vi "ResetTCPCommands&Responses_GIS Printer.vi"(8 "error in (no error)":errorcluster, 11 "GIS Printer In":refnum<class "GIS Printer.lvclass">) -> (0 "error out":errorcluster, 3 "GIS Printer Out":refnum<class "GIS Printer.lvclass">)   [LabVIEW 2022 SP3, in "GIS Printer.lvclass"]
uses:
  GIS Printer.lvclass
  GIS Printer.lvclass/GIS Printer.ctl
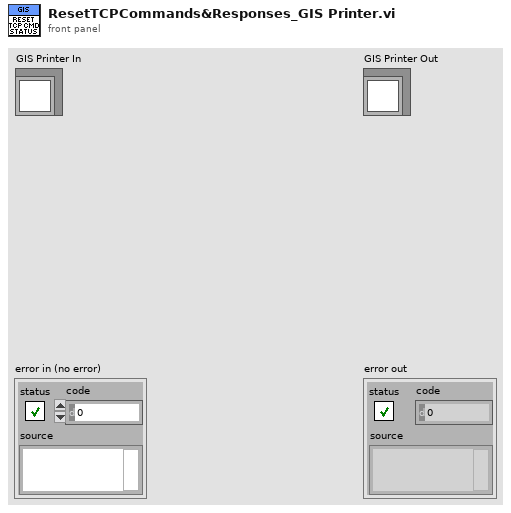
[diagram p1: front panel]
types:
  T1 = typedef "GIS Printer.lvclass/Private Data.ctl" = cluster{"UserEvents":T2, "All Dependencies":cluster{"Class References":refnum<class>[], "Class Names":string[]}, "PrinterConiguration":T3, "Status":T4, "GISHeadStatus":T5[], "HeadStatus":T6}
  T2 = typedef "GIS Printer.lvclass/UserEvents.ctl" = cluster{"API Incoming Event":refnum<user-event>, "API Executed Event":refnum<user-event>, "API Return Event":refnum<user-event>, "Status Changed Event":refnum<user-event>, "Abort":refnum<user-event>, "stop process":refnum<user-event>, "GISPollStatus":refnum<user-event>, "GISHeadStatus":refnum<user-event>}
  T3 = typedef "GIS Printer.lvclass/PrinterConfiguration--Cluster.ctl" = cluster{"IPAddress":string, "Move Stage on RTP Command?":bool, "Stage Move Position":string, "PH1-Prime Path":path, "PH2-Prime Path":path, "PH3-Prime Path":path, "PH4-Prime Path":path, "PH5-Prime Path":path, "PH6-Prime Path":path, "PrintScriptsFolder":path, "PurgeScriptsFolder":path, "StageScriptsFolder":path, "PH1-HeatOn Path":path, "PH2-HeatOn Path":path, "PH3-HeatOn Path":path, "PH4-HeatOn Path":path, "PH5-HeatOn Path":path, "PH6-HeatOn Path":path, "PH1-HeatOff Path":path, "PH2-HeatOff Path":path, "PH3-HeatOff Path":path, "PH4-HeatOff Path":path, "PH5-HeatOff Path":path, "PH6-HeatOff Path":path}
  T4 = typedef "GIS Printer.lvclass/Status Cluster.ctl" = cluster{"Command Status":variant, "TCP Commands & Responses":string[][], "Printer Busy?":bool}
  T5 = typedef "GIS Status--Cluster.ctl" = cluster{"HeadEnabled":bool, "SpitEnabled":bool, "HeaterEnabled":bool, "TargetTemperature":dbl, "CurrentTemperature":dbl}
  T6 = typedef "HeadEnableStatus--cluster.ctl" = cluster{"PH1_Enable":bool, "PH2_Enable":bool, "PH3_Enable":bool, "PH4_Enable":bool, "PH5_Enable":bool, "PH6_Enable":bool}
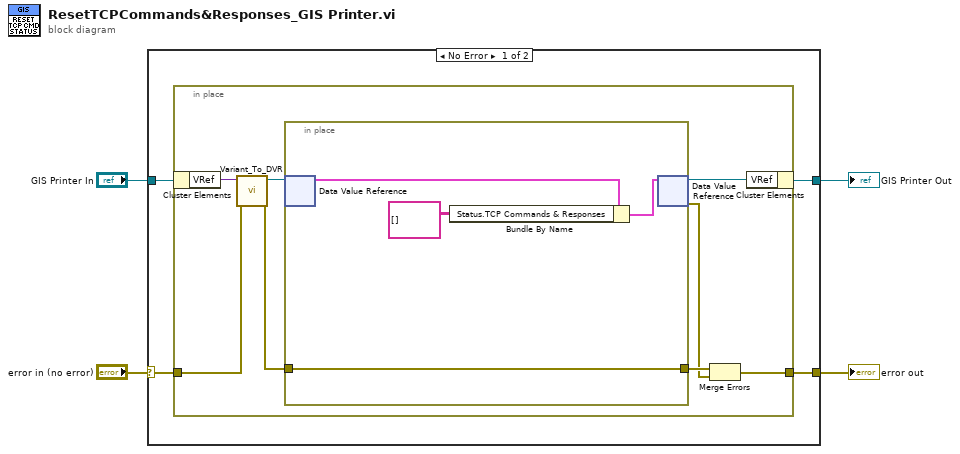
[diagram p0: block diagram]
diagram:
  n1 = case shown="No Error" "error in (no error)" {
    selector: "error in (no error)" -> [w5 w22]
    tunnel: [w7 w22] -> w3
    tunnel: [w8 w21] -> w1
    tunnel: "GIS Printer In" -> [w6 w21]
    frame No Error {
      n2 = in-place {
        in-place-border: w5 -> [w14]
        in-place-border: [w10] -> w7
        n3 = in-place-cluster #1(w6) -> ("VRef"=w16:variant)
        n4 = call "Variant_To_DVR.vi"("error in (no error)"=w14, "Variant"=w16) -> ("error out"=w13:errorcluster, "DVR"=w15:refnum<data-value>)  [unwired: 8 in]
        n5 = in-place {
          in-place-border: w13 -> [w18]
          in-place-border: [w18] -> w12
          n6 = in-place-dvr #2(w15) -> (w20:T1)  [unwired: 1 out]
          n7 = Bundle By Name(cluster=w20, "Status.TCP Commands & Responses"=string[][] []) -> (w19:T1)
          n8 = in-place-dvr #2(w19) -> (w9:refnum<data-value>, w11:errorcluster)
        }
        n9 = Merge Errors(w12, w11) -> (w10:errorcluster)
        n10 = in-place-cluster #1("VRef"=w9) -> (w8:refnum<class "GIS Printer.lvclass">)
      }
    }
    frame Error {
    }
  }
  "error out" <- w3
  "GIS Printer Out" <- w1
